vi "VM Monitor.vi"() -> ()   [LabVIEW 2010]
uses:
  <vilib>/Utility/sysdir.llb/System Directory Type.ctl
panel:
  in  "Reset":bool
  in  "Log":bool
  in  "Log to file":path
  in  "URL":refnum<visa-resource-name>="tcp://localhost"
  in  "Quit":bool
  in  "Duration":dbl[unit]=1000.0
  out "T":dbl[unit]=35.88999938964844 format="%_4g"
  out "gz":dbl[unit]=-0.004659709835278764 format="%_4p"
  out "gy":dbl[unit]=-0.022590839449213182 format="%_4p"
  out "gx":dbl[unit]=-0.019901542485926807 format="%_4p"
  out "az":dbl[unit]=0.00052925927734375 format="%_4g"
  out "ay":dbl[unit]=-0.00082588623046875 format="%_4g"
  out "ax":dbl[unit]=9.998315429687501e-05 format="%_4g"
  out "P":dbl[unit]=106140.01245117188 format="%_6g"
  out "BX":dbl[unit]=3.6740006401538853e-09 format="%_6g"
  out "BY":dbl[unit]=-5.247936037597656e-07 format="%_6g"
  out "BZ":dbl[unit]=-4.973549954223633e-07 format="%_6g"
  out "B":dbl[unit]=7.230379266504588e-07 format="%_6g"
  out "Field X":T1(graph)
  out "Field Y":T1(graph)
  out "Field Z":T1(graph)
  out "Field Total":T1(graph)
  out "ID":string="Twinleaf VM4 R4"
  in  "Bin":bool=TRUE
  out "XY Graph":T2(graph)
  # "VM Monitor"
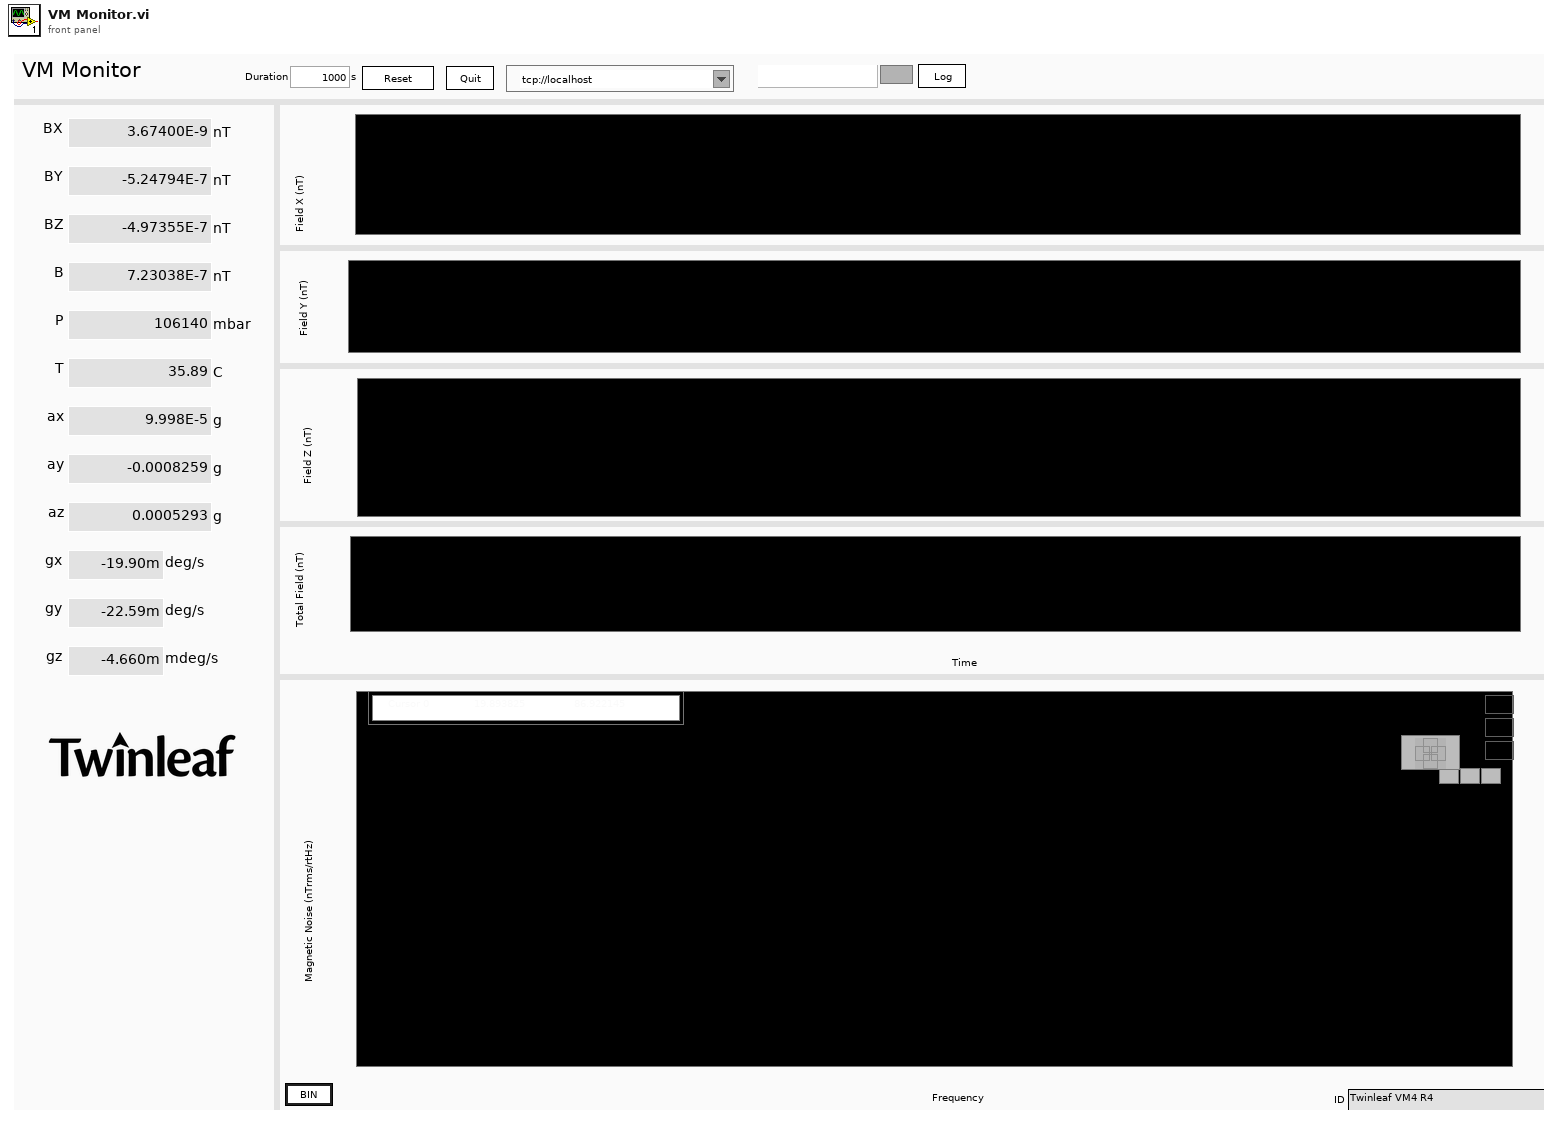
[diagram p1: front panel]
types:
  T1 = cluster{"start":dbl, "dt":dbl, "Timeseries":dbl[]}
  T2 = cluster{"Frequencies Binned":dbl[], "Spectrum Binned":dbl[]}[]
  T3 = cluster{"Awaiting REP":bool, "REQ ID":u32, "dstreams in":cluster{"id":u16, "timebase id":u16, "period":u32, "offset":u32, "sample number":u64, "total components":u16, "flags":u16, "components":cluster{"pstream id":u16, "flags":u16, "period":u32, "offset":u32}[]}[], "pstreams":cluster{"id":u16, "timebase_id":u16, "period":u32, "offset":u32, "fmt":i32, "flags":u16, "channels":u16, "type":u8, "name":string, "column names":string[], "title":string, "units":string}[], "timebases":cluster{"id":u16, "source":u16, "epoch":u32, "start time":u32, "period numerator (µs)":i32, "period denominator (µs)":u16, "flags":u16, "stability":u8, "source id":string}[]}
  T4 = typedef "System Directory Type.ctl" = i32
  T5 = cluster{"TS Connection":cluster{"Type":enum16{"Serial", "TCP", "UDP", "mUDP"}, "URL":refnum<visa-resource-name>, "TO":u32, "Addr":u32, "Port":i32, "TCP":refnum<k5>, "UDP":refnum<k16>, "Route":string}, "REQ":refnum<queue>, "REP":refnum<queue>}
  T6 = cluster{"start":dbl, "dt":dbl, "Timeseries":sgl[][]}
  T7 = cluster{"Awaiting REP":bool, "REQ ID":u32, "dstreams in":cluster{"id":u16, "timebase id":u16, "period":u32, "offset":u32, "sample number":u64, "total components":u16, "flags":u16, "components":cluster{"pstream id":u16, "flags":u16, "period":u32, "offset":u32}[]}[], "pstreams":cluster{"id":u16, "timebase_id":u16, "period":u32, "offset":u32, "fmt":i32, "flags":u16, "channels":u16, "type":u8, "name":string, "column names":string[], "title":string, "units":string}[], "timebases":cluster{"id":u16, "source":u16, "epoch":u32, "start time":u64, "period numerator (µs)":u32, "period denominator (µs)":u32, "flags":u32, "stability":sgl, "source id":string}[]}
  T8 = cluster{"dstream ID":u16, "Sample Number":u32, "Raw Data":string}
  T9 = cluster{"Awaiting REP":bool, "REQ ID":u32, "dstreams in":cluster{"id":u16, "timebase id":u16, "period":u32, "offset":u32, "sample number":u64, "total components":u16, "flags":u16, "components":cluster{"pstream id":u16, "flags":u16, "period":u32, "offset":u32}[]}[], "pstreams":cluster{"id":u16, "timebase_id":u16, "period":u32, "offset":u32, "fmt":i32, "flags":u16, "channels":u16, "type":u8, "name":string, "column names":string[], "title":string, "units":string}[], "timebases":cluster{"id":u16, "source":u8, "epoch":u8, "start time":u64, "period numerator (µs)":u32, "period denominator (µs)":u32, "flags":u32, "stability":sgl, "source id":string}[]}
  T10 = cluster{"TC Connection":cluster{"Type":enum16{"Serial", "TCP", "UDP", "mUDP"}, "URL":refnum<visa-resource-name>, "TO":u32, "Addr":u32, "Port":i32, "TCP":refnum<k5>, "UDP":refnum<k16>, "Route":string}, "REQ":refnum<queue>, "REP":refnum<queue>}
  T11 = cluster{"Name":string, "Waveform":cluster{"start":dbl, "dt":dbl, "Timeseries":dbl[][]}}[]
  T12 = cluster{"start":dbl, "dt":dbl, "Timeseries":dbl[][]}
  T13 = cluster{"Frequencies Binned":dbl[], "Spectrum Binned":dbl[]}
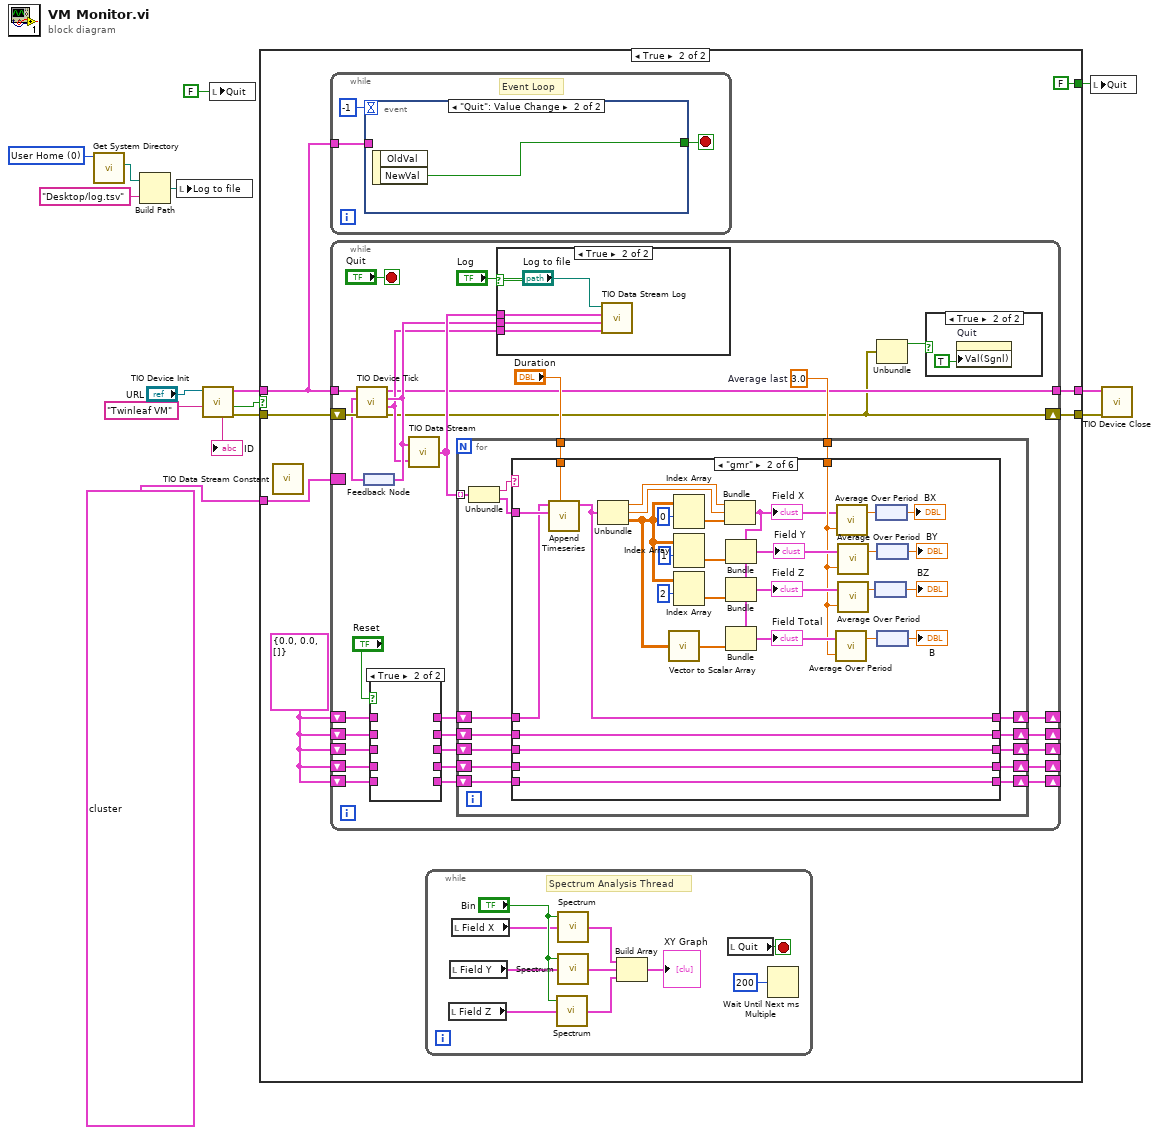
[diagram p0: block diagram]
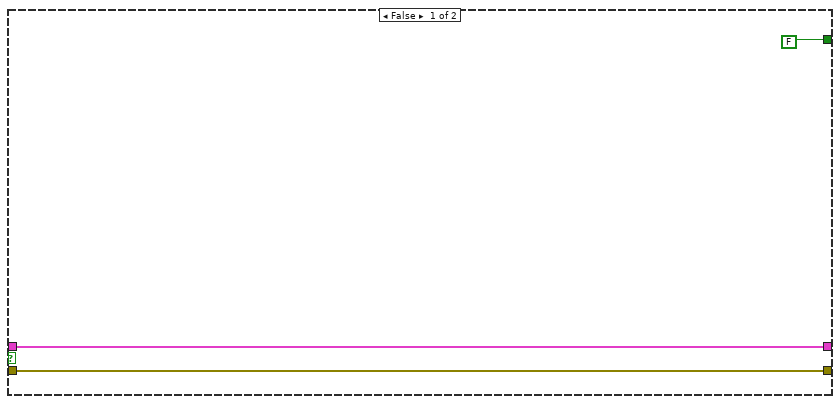
[diagram p2: hidden frame]
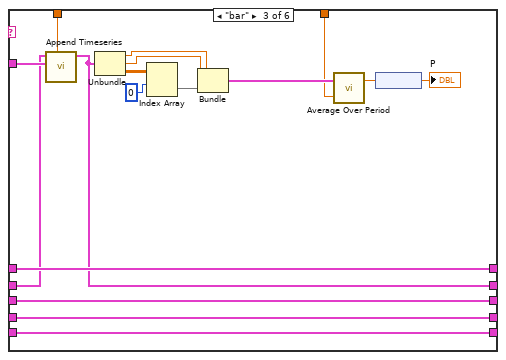
[diagram p6: hidden frame]
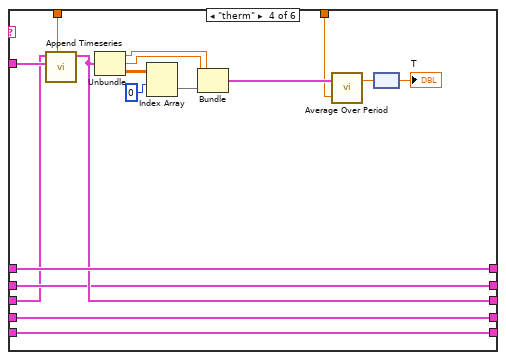
[diagram p7: hidden frame]
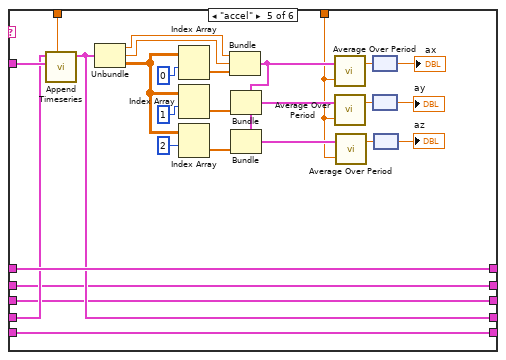
[diagram p8: hidden frame]
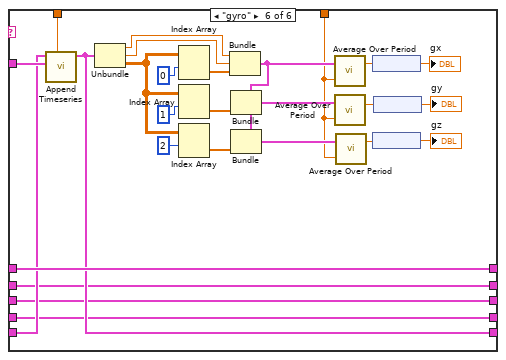
[diagram p9: hidden frame]
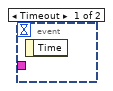
[diagram p11: hidden frame]
diagram:
  w9 = T4 0 items=["User Home"=0, "User Desktop"=1, "User Documents"=2, "User Application Data"=3, "User Preferences"=4, "User Temporary"=5, "Public Documents"=6, "Public Application Data"=7, "Public Preferences"=8, "Public Cache"=13, "System Core Libraries"=9, "System Installed Libraries"=10, "Application Files"=11, "Boot Volume Root"=12] ("system directory type")
  n1 = call <vilib>:"Get System Directory.vi"("system directory type"=w9) -> ("system directory"=w8:path)  [unwired: 10 in]
  n2 = Build Path(base path=w8, name or relative path="Desktop/log.tsv") -> (appended path=w6:path)
  n3 = local write "Log to file"(w6) -> ()
  n4 = call "TIO Device Init.vi"("ID"="Twinleaf VM" ("Prefix"), "URL"="URL") -> ("error out"=w14:errorcluster, "Connected"=w2:bool, "TIO"=w15:T5, "ID Verified"=→"ID":string)  [unwired: 5 in, 1 out]
  n5 = local write "Quit"(FALSE ("Kill")) -> ()
  n6 = case shown="True" w2 {
    tunnel: w15 -> [w17 w24]
    tunnel: w14 -> [w16 w25]
    tunnel: [FALSE FALSE ("Kill")] -> w10
    tunnel: [w17 w21] -> w4
    tunnel: [w16 w20] -> w5
    tunnel: T3 {"Awaiting REP"=FALSE, "REQ ID"=500, "dstreams in"=[{"id"=0, "timebase id"=1, "period"=4, "offset"=0, "sample number"=914806, "total components"=5, "flags"=1, "components"=[{"pstream id"=0, "flags"=0, "period"=1, "offset"=0}, {"pstream id"=1, "flags"=1, "period"=5, "offset"=0}, {"pstream id"=2, "flags"=1, "period"=5, "offset"=0}, {"pstream id"=3, "flags"=0, "period"=100, "offset"=0}, {"pstream id"=4, "flags"=0, "period"=100, "offset"=0}]}, {"id"=0, "timebase id"=0, "period"=0, "offset"=0, "sample number"=0, "total components"=0, "flags"=0, "components"=[]}, {"id"=0, "timebase id"=0, "period"=0, "offset"=0, "sample number"=0, "total components"=0, "flags"=0, "components"=[]}, {"id"=0, "timebase id"=0, "period"=0, "offset"=0, "sample number"=0, "total components"=0, "flags"=0, "components"=[]}, {"id"=0, "timebase id"=0, "period"=0, "offset"=0, "sample number"=0, "total components"=0, "flags"=0, "components"=[]}, {"id"=0, "timebase id"=0, "period"=0, "offset"=0, "sample number"=0, "total components"=0, "flags"=0, "components"=[]}, {"id"=0, "timebase id"=0, "period"=0, "offset"=0, "sample number"=0, "total components"=0, "flags"=0, "components"=[]}, {"id"=0, "timebase id"=0, "period"=0, "offset"=0, "sample number"=0, "total components"=0, "flags"=0, "components"=[]}, {"id"=0, "timebase id"=0, "period"=0, "offset"=0, "sample number"=0, "total components"=0, "flags"=0, "components"=[]}, {"id"=0, "timebase id"=0, "period"=0, "offset"=0, "sample number"=0, "total components"=0, "flags"=0, "components"=[]}, {"id"=0, "timebase id"=0, "period"=0, "offset"=0, "sample number"=0, "total components"=0, "flags"=0, "components"=[]}, {"id"=0, "timebase id"=0, "period"=0, "offset"=0, "sample number"=0, "total components"=0, "flags"=0, "components"=[]}, {"id"=0, "timebase id"=0, "period"=0, "offset"=0, "sample number"=0, "total components"=0, "flags"=0, "components"=[]}, {"id"=0, "timebase id"=0, "period"=0, "offset"=0, "sample number"=0, "total components"=0, "flags"=0, "components"=[]}, {"id"=0, "timebase id"=0, "period"=0, "offset"=0, "sample number"=0, "total components"=0, "flags"=0, "components"=[]}, {"id"=0, "timebase id"=0, "period"=0, "offset"=0, "sample number"=0, "total components"=0, "flags"=0, "components"=[]}, {"id"=0, "timebase id"=0, "period"=0, "offset"=0, "sample number"=0, "total components"=0, "flags"=0, "components"=[]}, {"id"=0, "timebase id"=0, "period"=0, "offset"=0, "sample number"=0, "total components"=0, "flags"=0, "components"=[]}, {"id"=0, "timebase id"=0, "period"=0, "offset"=0, "sample number"=0, "total components"=0, "flags"=0, "components"=[]}, {"id"=0, "timebase id"=0, "period"=0, "offset"=0, "sample number"=0, "total components"=0, "flags"=0, "components"=[]}, {"id"=0, "timebase id"=0, "period"=0, "offset"=0, "sample number"=0, "total components"=0, "flags"=0, "components"=[]}, {"id"=0, "timebase id"=0, "period"=0, "offset"=0, "sample number"=0, "total components"=0, "flags"=0, "components"=[]}, {"id"=0, "timebase id"=0, "period"=0, "offset"=0, "sample number"=0, "total components"=0, "flags"=0, "components"=[]}, {"id"=0, "timebase id"=0, "period"=0, "offset"=0, "sample number"=0, "total components"=0, "flags"=0, "components"=[]}, {"id"=0, "timebase id"=0, "period"=0, "offset"=0, "sample number"=0, "total components"=0, "flags"=0, "components"=[]}, {"id"=0, "timebase id"=0, "period"=0, "offset"=0, "sample number"=0, "total components"=0, "flags"=0, "components"=[]}, {"id"=0, "timebase id"=0, "period"=0, "offset"=0, "sample number"=0, "total components"=0, "flags"=0, "components"=[]}, {"id"=0, "timebase id"=0, "period"=0, "offset"=0, "sample number"=0, "total components"=0, "flags"=0, "components"=[]}, {"id"=0, "timebase id"=0, "period"=0, "offset"=0, "sample number"=0, "total components"=0, "flags"=0, "components"=[]}, {"id"=0, "timebase id"=0, "period"=0, "offset"=0, "sample number"=0, "total components"=0, "flags"=0, "components"=[]}, {"id"=0, "timebase id"=0, "period"=0, "offset"=0, "sample number"=0, "total components"=0, "flags"=0, "components"=[]}, {"id"=0, "timebase id"=0, "period"=0, "offset"=0, "sample number"=0, "total components"=0, "flags"=0, "components"=[]}], "pstreams"=[{"id"=0, "timebase_id"=1, "period"=1, "offset"=0, "fmt"=-1, "flags"=0, "channels"=3, "type"=66, "name"="gmr", "column names"=["x", "y", "z"], "title"="Vector magnetic field", "units"="nT"}, {"id"=1, "timebase_id"=1, "period"=8, "offset"=0, "fmt"=-1, "flags"=0, "channels"=3, "type"=66, "name"="accel", "column names"=["x", "y", "z"], "title"="Acceleration", "units"="m/s^2"}, {"id"=2, "timebase_id"=1, "period"=8, "offset"=0, "fmt"=-1, "flags"=0, "channels"=3, "type"=66, "name"="gyro", "column names"=["x", "y", "z"], "title"="Angular velocity", "units"="rad/s"}, {"id"=3, "timebase_id"=1, "period"=80, "offset"=0, "fmt"=-1, "flags"=0, "channels"=1, "type"=66, "name"="bar", "column names"=[""], "title"="Atmospheric pressure", "units"="mbar"}, {"id"=4, "timebase_id"=1, "period"=80, "offset"=0, "fmt"=-1, "flags"=0, "channels"=1, "type"=66, "name"="therm", "column names"=[""], "title"="Ambient temperature", "units"="C"}, {"id"=0, "timebase_id"=0, "period"=0, "offset"=0, "fmt"=0, "flags"=0, "channels"=0, "type"=0, "name"="", "column names"=[], "title"="", "units"=""}, {"id"=0, "timebase_id"=0, "period"=0, "offset"=0, "fmt"=0, "flags"=0, "channels"=0, "type"=0, "name"="", "column names"=[], "title"="", "units"=""}, {"id"=0, "timebase_id"=0, "period"=0, "offset"=0, "fmt"=0, "flags"=0, "channels"=0, "type"=0, "name"="", "column names"=[], "title"="", "units"=""}, {"id"=0, "timebase_id"=0, "period"=0, "offset"=0, "fmt"=0, "flags"=0, "channels"=0, "type"=0, "name"="", "column names"=[], "title"="", "units"=""}, {"id"=0, "timebase_id"=0, "period"=0, "offset"=0, "fmt"=0, "flags"=0, "channels"=0, "type"=0, "name"="", "column names"=[], "title"="", "units"=""}, {"id"=0, "timebase_id"=0, "period"=0, "offset"=0, "fmt"=0, "flags"=0, "channels"=0, "type"=0, "name"="", "column names"=[], "title"="", "units"=""}, {"id"=0, "timebase_id"=0, "period"=0, "offset"=0, "fmt"=0, "flags"=0, "channels"=0, "type"=0, "name"="", "column names"=[], "title"="", "units"=""}, {"id"=0, "timebase_id"=0, "period"=0, "offset"=0, "fmt"=0, "flags"=0, "channels"=0, "type"=0, "name"="", "column names"=[], "title"="", "units"=""}, {"id"=0, "timebase_id"=0, "period"=0, "offset"=0, "fmt"=0, "flags"=0, "channels"=0, "type"=0, "name"="", "column names"=[], "title"="", "units"=""}, {"id"=0, "timebase_id"=0, "period"=0, "offset"=0, "fmt"=0, "flags"=0, "channels"=0, "type"=0, "name"="", "column names"=[], "title"="", "units"=""}, {"id"=0, "timebase_id"=0, "period"=0, "offset"=0, "fmt"=0, "flags"=0, "channels"=0, "type"=0, "name"="", "column names"=[], "title"="", "units"=""}, {"id"=32768, "timebase_id"=1, "period"=1, "offset"=0, "fmt"=-1, "flags"=0, "channels"=3, "type"=66, "name"="_gmr.raw", "column names"=["x", "y", "z"], "title"="Vector magnetic field", "units"="nT"}, {"id"=32769, "timebase_id"=1, "period"=8, "offset"=0, "fmt"=-1, "flags"=0, "channels"=3, "type"=66, "name"="_accel.raw", "column names"=["x", "y", "z"], "title"="Acceleration", "units"="m/s^2"}, {"id"=32770, "timebase_id"=1, "period"=8, "offset"=0, "fmt"=-1, "flags"=0, "channels"=3, "type"=66, "name"="_gyro.raw", "column names"=["x", "y", "z"], "title"="Angular velocity", "units"="rad/s"}, {"id"=32771, "timebase_id"=1, "period"=80, "offset"=0, "fmt"=-1, "flags"=0, "channels"=1, "type"=66, "name"="_bar.raw", "column names"=[""], "title"="Atmospheric pressure", "units"="mbar"}, {"id"=32772, "timebase_id"=1, "period"=80, "offset"=0, "fmt"=-1, "flags"=0, "channels"=1, "type"=66, "name"="_therm.raw", "column names"=[""], "title"="Ambient temperature", "units"="C"}, {"id"=32773, "timebase_id"=0, "period"=1, "offset"=0, "fmt"=-1, "flags"=0, "channels"=1, "type"=66, "name"="_cpu.raw", "column names"=[""], "title"="CPU load", "units"="%"}, {"id"=32774, "timebase_id"=0, "period"=1, "offset"=0, "fmt"=-1, "flags"=0, "channels"=1, "type"=66, "name"="cpu", "column names"=[""], "title"="CPU load", "units"="%"}, {"id"=0, "timebase_id"=0, "period"=0, "offset"=0, "fmt"=0, "flags"=0, "channels"=0, "type"=0, "name"="", "column names"=[], "title"="", "units"=""}, {"id"=0, "timebase_id"=0, "period"=0, "offset"=0, "fmt"=0, "flags"=0, "channels"=0, "type"=0, "name"="", "column names"=[], "title"="", "units"=""}, {"id"=0, "timebase_id"=0, "period"=0, "offset"=0, "fmt"=0, "flags"=0, "channels"=0, "type"=0, "name"="", "column names"=[], "title"="", "units"=""}, {"id"=0, "timebase_id"=0, "period"=0, "offset"=0, "fmt"=0, "flags"=0, "channels"=0, "type"=0, "name"="", "column names"=[], "title"="", "units"=""}, {"id"=0, "timebase_id"=0, "period"=0, "offset"=0, "fmt"=0, "flags"=0, "channels"=0, "type"=0, "name"="", "column names"=[], "title"="", "units"=""}, {"id"=0, "timebase_id"=0, "period"=0, "offset"=0, "fmt"=0, "flags"=0, "channels"=0, "type"=0, "name"="", "column names"=[], "title"="", "units"=""}, {"id"=0, "timebase_id"=0, "period"=0, "offset"=0, "fmt"=0, "flags"=0, "channels"=0, "type"=0, "name"="", "column names"=[], "title"="", "units"=""}, {"id"=0, "timebase_id"=0, "period"=0, "offset"=0, "fmt"=0, "flags"=0, "channels"=0, "type"=0, "name"="", "column names"=[], "title"="", "units"=""}, {"id"=0, "timebase_id"=0, "period"=0, "offset"=0, "fmt"=0, "flags"=0, "channels"=0, "type"=0, "name"="", "column names"=[], "title"="", "units"=""}], "timebases"=[{"id"=0, "source"=513, "epoch"=0, "start time"=0, "period numerator (µs)"=100000000, "period denominator (µs)"=1000, "flags"=0, "stability"=1, "source id"="\u0000\u0000\u0000¬Å'7\u0001\u0000\u0000\u0000B\u0000!\u0000\u0011P6W462 "}, {"id"=1, "source"=513, "epoch"=194250488, "start time"=0, "period numerator (µs)"=1250000, "period denominator (µs)"=1000, "flags"=0, "stability"=1, "source id"="\u0000\u0000\u0000¬Å'7\u0001\u0000\u0000\u0000B\u0000!\u0000\u0011P6W462 "}, {"id"=0, "source"=0, "epoch"=0, "start time"=0, "period numerator (µs)"=0, "period denominator (µs)"=0, "flags"=0, "stability"=0, "source id"=""}, {"id"=0, "source"=0, "epoch"=0, "start time"=0, "period numerator (µs)"=0, "period denominator (µs)"=0, "flags"=0, "stability"=0, "source id"=""}, {"id"=0, "source"=0, "epoch"=0, "start time"=0, "period numerator (µs)"=0, "period denominator (µs)"=0, "flags"=0, "stability"=0, "source id"=""}, {"id"=0, "source"=0, "epoch"=0, "start time"=0, "period numerator (µs)"=0, "period denominator (µs)"=0, "flags"=0, "stability"=0, "source id"=""}, {"id"=0, "source"=0, "epoch"=0, "start time"=0, "period numerator (µs)"=0, "period denominator (µs)"=0, "flags"=0, "stability"=0, "source id"=""}, {"id"=0, "source"=0, "epoch"=0, "start time"=0, "period numerator (µs)"=0, "period denominator (µs)"=0, "flags"=0, "stability"=0, "source id"=""}, {"id"=0, "source"=0, "epoch"=0, "start time"=0, "period numerator (µs)"=0, "period denominator (µs)"=0, "flags"=0, "stability"=0, "source id"=""}, {"id"=0, "source"=0, "epoch"=0, "start time"=0, "period numerator (µs)"=0, "period denominator (µs)"=0, "flags"=0, "stability"=0, "source id"=""}, {"id"=0, "source"=0, "epoch"=0, "start time"=0, "period numerator (µs)"=0, "period denominator (µs)"=0, "flags"=0, "stability"=0, "source id"=""}, {"id"=0, "source"=0, "epoch"=0, "start time"=0, "period numerator (µs)"=0, "period denominator (µs)"=0, "flags"=0, "stability"=0, "source id"=""}, {"id"=0, "source"=0, "epoch"=0, "start time"=0, "period numerator (µs)"=0, "period denominator (µs)"=0, "flags"=0, "stability"=0, "source id"=""}, {"id"=0, "source"=0, "epoch"=0, "start time"=0, "period numerator (µs)"=0, "period denominator (µs)"=0, "flags"=0, "stability"=0, "source id"=""}, {"id"=0, "source"=0, "epoch"=0, "start time"=0, "period numerator (µs)"=0, "period denominator (µs)"=0, "flags"=0, "stability"=0, "source id"=""}, {"id"=0, "source"=0, "epoch"=0, "start time"=0, "period numerator (µs)"=0, "period denominator (µs)"=0, "flags"=0, "stability"=0, "source id"=""}, {"id"=0, "source"=0, "epoch"=0, "start time"=0, "period numerator (µs)"=0, "period denominator (µs)"=0, "flags"=0, "stability"=0, "source id"=""}, {"id"=0, "source"=0, "epoch"=0, "start time"=0, "period numerator (µs)"=0, "period denominator (µs)"=0, "flags"=0, "stability"=0, "source id"=""}, {"id"=0, "source"=0, "epoch"=0, "start time"=0, "period numerator (µs)"=0, "period denominator (µs)"=0, "flags"=0, "stability"=0, "source id"=""}, {"id"=0, "source"=0, "epoch"=0, "start time"=0, "period numerator (µs)"=0, "period denominator (µs)"=0, "flags"=0, "stability"=0, "source id"=""}, {"id"=0, "source"=0, "epoch"=0, "start time"=0, "period numerator (µs)"=0, "period denominator (µs)"=0, "flags"=0, "stability"=0, "source id"=""}, {"id"=0, "source"=0, "epoch"=0, "start time"=0, "period numerator (µs)"=0, "period denominator (µs)"=0, "flags"=0, "stability"=0, "source id"=""}, {"id"=0, "source"=0, "epoch"=0, "start time"=0, "period numerator (µs)"=0, "period denominator (µs)"=0, "flags"=0, "stability"=0, "source id"=""}, {"id"=0, "source"=0, "epoch"=0, "start time"=0, "period numerator (µs)"=0, "period denominator (µs)"=0, "flags"=0, "stability"=0, "source id"=""}, {"id"=0, "source"=0, "epoch"=0, "start time"=0, "period numerator (µs)"=0, "period denominator (µs)"=0, "flags"=0, "stability"=0, "source id"=""}, {"id"=0, "source"=0, "epoch"=0, "start time"=0, "period numerator (µs)"=0, "period denominator (µs)"=0, "flags"=0, "stability"=0, "source id"=""}, {"id"=0, "source"=0, "epoch"=0, "start time"=0, "period numerator (µs)"=0, "period denominator (µs)"=0, "flags"=0, "stability"=0, "source id"=""}, {"id"=0, "source"=0, "epoch"=0, "start time"=0, "period numerator (µs)"=0, "period denominator (µs)"=0, "flags"=0, "stability"=0, "source id"=""}, {"id"=0, "source"=0, "epoch"=0, "start time"=0, "period numerator (µs)"=0, "period denominator (µs)"=0, "flags"=0, "stability"=0, "source id"=""}, {"id"=0, "source"=0, "epoch"=0, "start time"=0, "period numerator (µs)"=0, "period denominator (µs)"=0, "flags"=0, "stability"=0, "source id"=""}, {"id"=0, "source"=0, "epoch"=0, "start time"=0, "period numerator (µs)"=0, "period denominator (µs)"=0, "flags"=0, "stability"=0, "source id"=""}, {"id"=0, "source"=0, "epoch"=0, "start time"=0, "period numerator (µs)"=0, "period denominator (µs)"=0, "flags"=0, "stability"=0, "source id"=""}]} ("TIO State") -> [_ w19]
    frame False {
    }
    frame True {
      w22 = T6 {"start"=0.0, "dt"=0.0, "Timeseries"=[]}
      n7 = call "TIO Data Stream Constant.vi"() -> ()  [unwired: 1 out]
      n8 = while {
        tunnel: w24 -> [w205]
        stop <- w204 stop-if-true
        # "Event Loop"
        n9 = event shown="[1] \"Quit\": Value Change" {
          selector: _ -> [_ _]
          dyn-events: _ -> [_ _]
          timeout: -1 -> [_ _]
          tunnel: w205 -> [_ _]
          tunnel: [_ w207] -> w204
          event Timeout {
            n10 = event-data() -> ()  [unwired: 1 in, 1 out]
          }
          event "Quit": Value Change {
            n11 = event-data() -> ("NewVal"=w207:bool)  [unwired: 1 in, 1 out]
          }
        }
      }
      n12 = while {
        tunnel: w24 -> [w54]
        shift-right: [w50] -> _
        shift-left: w22 -> [w38]
        shift-right: [w47] -> _
        shift-left: w22 -> [w37]
        shift-right: [w46] -> _
        shift-left: w22 -> [w36]
        shift-right: [w45] -> _
        shift-left: w22 -> [w35]
        shift-right: [w44] -> _
        shift-left: w22 -> [w34]
        border: w19 -> [_]
        tunnel: [w28] -> w21
        shift-right: [w27] -> w20
        shift-left: w25 -> [w53]
        stop <- "Quit" stop-if-true
        w49 = dbl[unit] 3.0  # Average last
        n13 = feedback #1() -> (w43:T7)
        n14 = call "TIO Device Tick.vi"("Error in"=w53, "TIO State"=w43, "TIO"=w54) -> ("Error out"=w27:errorcluster, "Data Out"=w40:T8, "TIO State"=w41:T9, "TIO"=w28:T10)  [unwired: 5 in]
        n15 = feedback-in #1(w41) -> ()
        n16 = case shown="True" "Reset" {
          tunnel: w38 -> [w60 _]
          tunnel: w37 -> [w59 _]
          tunnel: w36 -> [w58 _]
          tunnel: w35 -> [w57 _]
          tunnel: w34 -> [w56 _]
          tunnel: [w56 _] -> w33
          tunnel: [w57 _] -> w32
          tunnel: [w58 _] -> w31
          tunnel: [w59 _] -> w30
          tunnel: [w60 _] -> w29
          frame False {
          }
          frame True {
          }
        }
        n17 = call "TIO Data Stream.vi"("Raw Data"=w40, "TIO State"=w41) -> ("Data Out"=w42:T11)
        n18 = for {
          tunnel: "Duration" -> [w75]
          tunnel: w49 -> [w72]
          tunnel: w42 -> [w63] mode=indexing
          shift-right: [w74] -> w50
          shift-left: w29 -> [w73]
          shift-right: [w71] -> w47
          shift-left: w30 -> [w70]
          shift-right: [w69] -> w46
          shift-left: w31 -> [w68]
          shift-right: [w67] -> w45
          shift-left: w32 -> [w66]
          shift-right: [w65] -> w44
          shift-left: w33 -> [w64]
          n19 = Unbundle(w63) -> ("Name"=w62:string, "Waveform"=w61:T12)
          n20 = case shown="\"gmr\"" w62 {
            tunnel: w75 -> [_ w111 w128 w145 w172 w199]
            tunnel: w72 -> [_ w92 w117 w135 w151 w184]
            tunnel: w61 -> [_ w87 w121 w139 w155 w188]
            tunnel: [w80 w86 w120 w138 w152 w185] -> w74
            tunnel: w73 -> [w80 w85 w120 w138 w152 w185]
            tunnel: [w79 w84 w116 w132 w148 w175] -> w71
            tunnel: w70 -> [w79 w84 w115 w132 w148 w175]
            tunnel: [w78 w83 w114 w133 w147 w174] -> w69
            tunnel: w68 -> [w78 w83 w114 w131 w147 w174]
            tunnel: [w77 w82 w113 w130 w150 w173] -> w67
            tunnel: w66 -> [w77 w82 w113 w130 w149 w173]
            tunnel: [w76 w81 w112 w129 w146 w177] -> w65
            tunnel: w64 -> [w76 w81 w112 w129 w146 w176]
            frame Default {
            }
            frame "gmr" {
              n21 = call "Append Timeseries.vi"("Duration"=w111, "In New"=w87, "In Old"=w85) -> ("Appended"=w86:T12)  [unwired: 8 in]
              n22 = Unbundle(w86) -> ("start"=w110:dbl, "dt"=w91:dbl, "Timeseries"=w89:dbl[][])
              n23 = call "Vector to Scalar Array.vi"("Three axis vector"=w89) -> ("Total field"=w88:dbl[])
              n24 = Index Array(array=w89, index (row)=0 ("disabled index (col)")) -> (element=w106:dbl[])  [unwired: 1 in]
              n25 = Index Array(array=w89, index (row)=1 ("disabled index (col)")) -> (element=w105:dbl[])  [unwired: 1 in]
              n26 = Index Array(array=w89, index (row)=2 ("disabled index (col)")) -> (element=w104:dbl[])  [unwired: 1 in]
              n27 = Bundle("start"=w110, "dt"=w91, "Timeseries"=w106) -> (w90:T1)  [unwired: 1 in]
              "Field X" <- w90
              n28 = Bundle(cluster=w90, "Timeseries"=w105) -> (w101:T1)  [unwired: 2 in]
              "Field Y" <- w101
              n29 = Bundle(cluster=w90, "Timeseries"=w104) -> (w100:T1)  [unwired: 2 in]
              "Field Z" <- w100
              n30 = Bundle(cluster=w90, "Timeseries"=w88) -> (w99:T1)  [unwired: 2 in]
              "Field Total" <- w99
              n31 = call "Average Over Period.vi"("Period"=w92, "Cluster"=w99) -> ("Average"=w94:dbl)  [unwired: 1 in]
              n32 = call "Average Over Period.vi"("Period"=w92, "Cluster"=w90) -> ("Average"=w103:dbl)  [unwired: 1 in]
              n33 = call "Average Over Period.vi"("Period"=w92, "Cluster"=w101) -> ("Average"=w98:dbl)  [unwired: 1 in]
              n34 = call "Average Over Period.vi"("Period"=w92, "Cluster"=w100) -> ("Average"=w96:dbl)  [unwired: 1 in]
              n35 = node(w96) -> (→"BZ":dbl[unit])
              n36 = node(w103) -> (→"BX":dbl[unit])
              n37 = node(w98) -> (→"BY":dbl[unit])
              n38 = node(w94) -> (→"B":dbl[unit])
            }
            frame "bar" {
              n39 = call "Append Timeseries.vi"("Duration"=w128, "In New"=w121, "In Old"=w115) -> ("Appended"=w116:T12)  [unwired: 8 in]
              n40 = Unbundle(w116) -> ("start"=w126:dbl, "dt"=w127:dbl, "Timeseries"=w119:dbl[][])
              n41 = Index Array(array=w119, index (row)=0 ("disabled index (col)")) -> (element=w124:dbl[])  [unwired: 1 in]
              n42 = Bundle("start"=w126, "dt"=w127, "Timeseries"=w124) -> (w118:T1)  [unwired: 1 in]
              n43 = call "Average Over Period.vi"("Period"=w117, "Cluster"=w118) -> ("Average"=w122:dbl)  [unwired: 1 in]
              n44 = node(w122) -> (→"P":dbl[unit])
            }
            frame "therm" {
              n45 = call "Append Timeseries.vi"("Duration"=w145, "In New"=w139, "In Old"=w131) -> ("Appended"=w133:T12)  [unwired: 8 in]
              n46 = Unbundle(w133) -> ("start"=w143:dbl, "dt"=w144:dbl, "Timeseries"=w137:dbl[][])
              n47 = Index Array(array=w137, index (row)=0 ("disabled index (col)")) -> (element=w141:dbl[])  [unwired: 1 in]
              n48 = Bundle("start"=w143, "dt"=w144, "Timeseries"=w141) -> (w136:T1)  [unwired: 1 in]
              n49 = call "Average Over Period.vi"("Period"=w135, "Cluster"=w136) -> ("Average"=w140:dbl)  [unwired: 1 in]
              n50 = node(w140) -> (→"T":dbl[unit])
            }
            frame "accel" {
              n51 = call "Append Timeseries.vi"("Duration"=w172, "In New"=w155, "In Old"=w149) -> ("Appended"=w150:T12)  [unwired: 8 in]
              n52 = Unbundle(w150) -> ("start"=w170:dbl, "dt"=w171:dbl, "Timeseries"=w154:dbl[][])
              n53 = Index Array(array=w154, index (row)=0 ("disabled index (col)")) -> (element=w167:dbl[])  [unwired: 1 in]
              n54 = Index Array(array=w154, index (row)=1 ("disabled index (col)")) -> (element=w166:dbl[])  [unwired: 1 in]
              n55 = Index Array(array=w154, index (row)=2 ("disabled index (col)")) -> (element=w163:dbl[])  [unwired: 1 in]
              n56 = Bundle("start"=w170, "dt"=w171, "Timeseries"=w167) -> (w153:T1)  [unwired: 1 in]
              n57 = Bundle(cluster=w153, "Timeseries"=w166) -> (w164:T1)  [unwired: 2 in]
              n58 = Bundle(cluster=w153, "Timeseries"=w163) -> (w161:T1)  [unwired: 2 in]
              n59 = call "Average Over Period.vi"("Period"=w151, "Cluster"=w153) -> ("Average"=w162:dbl)  [unwired: 1 in]
              n60 = call "Average Over Period.vi"("Period"=w151, "Cluster"=w164) -> ("Average"=w159:dbl)  [unwired: 1 in]
              n61 = call "Average Over Period.vi"("Period"=w151, "Cluster"=w161) -> ("Average"=w158:dbl)  [unwired: 1 in]
              n62 = node(w162) -> (→"ax":dbl[unit])
              n63 = node(w159) -> (→"ay":dbl[unit])
              n64 = node(w158) -> (→"az":dbl[unit])
            }
            frame "gyro" {
              n65 = call "Append Timeseries.vi"("Duration"=w199, "In New"=w188, "In Old"=w176) -> ("Appended"=w177:T12)  [unwired: 8 in]
              n66 = Unbundle(w177) -> ("start"=w197:dbl, "dt"=w198:dbl, "Timeseries"=w187:dbl[][])
              n67 = Index Array(array=w187, index (row)=0 ("disabled index (col)")) -> (element=w194:dbl[])  [unwired: 1 in]
              n68 = Index Array(array=w187, index (row)=1 ("disabled index (col)")) -> (element=w193:dbl[])  [unwired: 1 in]
              n69 = Index Array(array=w187, index (row)=2 ("disabled index (col)")) -> (element=w190:dbl[])  [unwired: 1 in]
              n70 = Bundle("start"=w197, "dt"=w198, "Timeseries"=w194) -> (w186:T1)  [unwired: 1 in]
              n71 = Bundle(cluster=w186, "Timeseries"=w193) -> (w191:T1)  [unwired: 2 in]
              n72 = Bundle(cluster=w186, "Timeseries"=w190) -> (w189:T1)  [unwired: 2 in]
              n73 = call "Average Over Period.vi"("Period"=w184, "Cluster"=w186) -> ("Average"=w180:dbl)  [unwired: 1 in]
              n74 = call "Average Over Period.vi"("Period"=w184, "Cluster"=w191) -> ("Average"=w179:dbl)  [unwired: 1 in]
              n75 = call "Average Over Period.vi"("Period"=w184, "Cluster"=w189) -> ("Average"=w178:dbl)  [unwired: 1 in]
              n76 = node(w180) -> (→"gx":dbl[unit])
              n77 = node(w178) -> (→"gz":dbl[unit])
              n78 = node(w179) -> (→"gy":dbl[unit])
            }
          }
        }
        n79 = case shown="True" "Log" {
          tunnel: w42 -> [_ w201]
          tunnel: w41 -> [_ w202]
          tunnel: w40 -> [_ w200]
          frame False {
          }
          frame True {
            n80 = call "TIO Data Stream Log.vi"(8:"Data Out"=w200, "TIO State"=w202, 10:"Data Out"=w201, "Log to file"="Log to file") -> ()  [unwired: 8 in]
          }
        }
        n81 = Unbundle(w27) -> ("status"=w26:bool)  [unwired: 2 out]
        n82 = case shown="True" w26 {
          frame False {
          }
          frame True {
            n83 = property on="Quit" class="Bool (strict)"("Val(Sgnl)"=TRUE ("Value (Signaling)")) -> ()  [unwired: 2 in, 2 out]
          }
        }
      }
      n84 = while {
        stop <- w211 stop-if-true
        # "Spectrum Analysis Thread"
        n85 = local read "Field Z"() -> (w208:T1)
        n86 = local read "Field Y"() -> (w209:T1)
        n87 = local read "Field X"() -> (w210:T1)
        n88 = call "Spectrum.vi"("Waveform 1"=w208, "Binning"="Bin") -> ("Cluster"=w213:T13)  [unwired: 3 in]
        n89 = call "Spectrum.vi"("Waveform 1"=w210, "Binning"="Bin") -> ("Cluster"=w215:T13)  [unwired: 3 in]
        n90 = call "Spectrum.vi"("Waveform 1"=w209, "Binning"="Bin") -> ("Cluster"=w214:T13)  [unwired: 3 in]
        n91 = Build Array(w215, w214, w213) -> (→"XY Graph":T2)
        n92 = local read "Quit"() -> (w211:bool)
        n93 = Wait Until Next ms Multiple(millisecond multiple=u32 200) -> ()  [unwired: 1 out]
      }
    }
  }
  n94 = local write "Quit"(w10) -> ()
  n95 = call "TIO Device Close.vi"("Error in"=w5, "TIO"=w4) -> ()  [unwired: 10 in]
